vi "arange.vi"(9 "Number of pixels":i32, 10 "end":dbl, 11 "begin":dbl) -> (3 "数组":dbl[](array[numeric]))   [LabVIEW 2013]
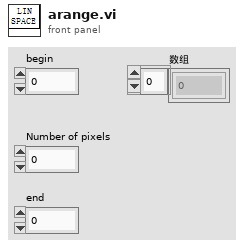
[diagram p1: front panel]
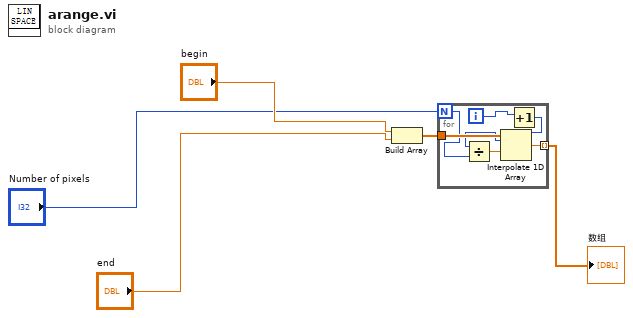
[diagram p0: block diagram]
diagram:
  n1 = Build Array("begin", "end") -> (w1:dbl[])
  n2 = for {
    N: "Number of pixels" -> [w8]
    tunnel: [w11] -> w2 mode=indexing
    tunnel: w1 -> [w10]
    i -> [w7]
    n3 = Increment(x=w7) -> (x+1=w6:i32)
    n4 = Divide(x=w6, y=w8) -> (x/y=w9:dbl)
    n5 = Interpolate 1D Array(1:w9, 2:w10) -> (0:w11:dbl)
  }
  "数组" <- w2
